vi "KE6517_Test.vi"(8 "error in (no error)":errorcluster, 11 "KE6517 in":refnum<class "KE6517.lvclass">) -> (0 "error out":errorcluster, 3 "KE6517 out":refnum<class "KE6517.lvclass">)   [LabVIEW 2013, in "KE6517.lvclass"]
uses:
  KE6517.lvclass
  <vilib>/Platform/TimedLoop/XDataNode/timing_clust.ctl
  <vilib>/Platform/TimedLoop/XDataNode/nitl_modes.ctl
  <vilib>/Platform/TimedLoop/XDataNode/wakeup.ctl
  InstrumentSetup.vi
  <vilib>/platform/TimedLoop/XDataNode/XDataNode.xnode
  <vilib>/Platform/TimedLoop/XDataNode/XDNodeRunTimeDep.lvlib
  InstrControl.lvclass
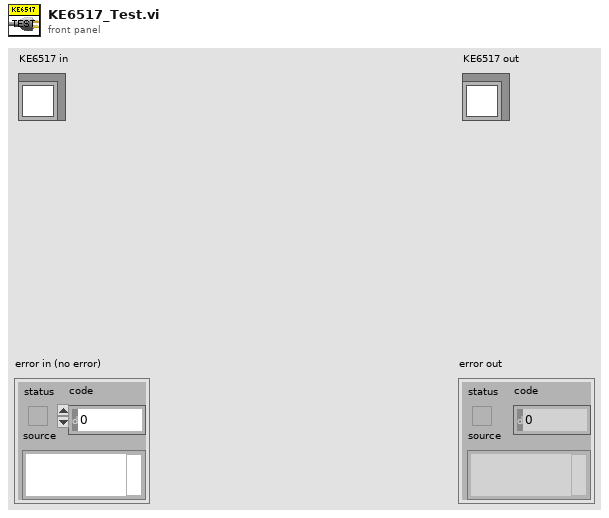
[diagram p1: front panel]
types:
  T1 = cluster{"KE 2410":cluster{"Instrument name":string, "address":refnum<visa-resource-name>, "Instrument type":u16}, "KE 6517":cluster{"Instrument name":string, "address":refnum<visa-resource-name>, "Instrument type":u16}, "KE 487":cluster{"Instrument name":string, "address":refnum<visa-resource-name>, "Instrument type":u16}, "KE 236":cluster{"Instrument name":string, "address":refnum<visa-resource-name>, "Instrument type":u16}, "WK 6440B":cluster{"Instrument name":string, "address":refnum<visa-resource-name>, "Instrument type":u16}, "WK 6425":cluster{"Instrument name":string, "address":refnum<visa-resource-name>, "Instrument type":u16}, "Pickering Matrix":cluster{"Instrument name":string, "address":refnum<visa-resource-name>, "Instrument type":u16}, "KE 2000":cluster{"Instrument name":string, "address":refnum<visa-resource-name>, "Instrument type":u16}, "KE3706A Switching":cluster{"Instrument name":string, "address":refnum<visa-resource-name>, "Instrument type":u16}}
  T2 = cluster{"Current Limit":u16, "KE6517":refnum<class "KE6517.lvclass">}
  T3 = typedef "XDNodeRunTimeDep.lvlib/timing_clust.ctl" = cluster{"Expected End [f-1]":u64, "Actual End [f-1]":u64, "Finished Late? [f-1]":bool, "Expected End [i-1]":u64, "Actual End [i-1]":u64, "Finished Late? [i-1]":bool, "Expected Start [i]":u64, "Actual Start [i]":u64, "Expected Start [f]":u64, "Actual Start [f]":u64, "Source Name":string, "Structure Name":string, "Period":i64, "Deadline":i64, "Offset":i64, "Start":i64, "Priority":i32, "Timeout":i32, "Mode":T4, "Wakeup Reason":T5, "Error":errorcluster, "Source Type":string, "Secondary Source Type":string, "Global End Time":u64, "Global Start Time":u64, "Frame Duration":u64, "Iteration Duration":u64, "Assigned CPU":i32, "I/O Scan Engine Mode":u32}
  T4 = typedef "XDNodeRunTimeDep.lvlib/nitl_modes.ctl" = enum32{"No Change", "Process missed periods, maintain original phase", "Discard missed periods, maintain original phase", "Process missed periods, ignore original phase", "Discard missed periods, ignore original phase"}
  T5 = typedef "XDNodeRunTimeDep.lvlib/wakeup.ctl" = enum32{"Normal", "Aborted", "Asynchronous wakeup", "Timing source error", "Timed loop error", "Timeout"}
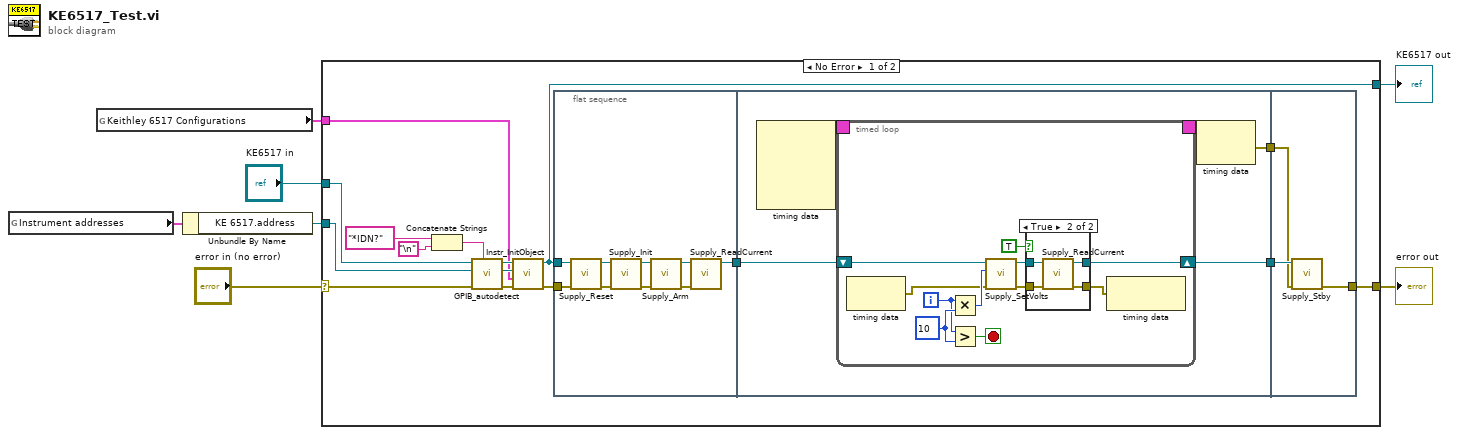
[diagram p0: block diagram]
diagram:
  n1 = global read "InstrumentSetup.vi" "Instrument addresses"() -> (w3:T1)
  n2 = global read "InstrumentSetup.vi" "Keithley 6517 Configurations"() -> (w1:T2)
  n3 = Unbundle By Name(w3) -> ("KE 6517.address"=w2:refnum<visa-resource-name>)
  n4 = case shown="No Error" "error in (no error)" {
    selector: "error in (no error)" -> [w18 w67]
    tunnel: [w20 w67] -> w6
    tunnel: [w16 w66] -> w4
    tunnel: "KE6517 in" -> [w14 w66]
    tunnel: w2 -> [w12 _]
    tunnel: w1 -> [w11 _]
    frame No Error {
      n5 = Concatenate Strings("*IDN?" ("regular expression"), "\n") -> (w9:string)
      n6 = call-dynamic "GPIB_autodetect.vi"("ID command"=w9, "error in (no error)"=w18, "Instrument address in"=w12, "InstrControl in"=w14) -> ("error out"=w19:errorcluster, "Instrument address out"=w13:refnum<visa-resource-name>, "InstrControl out"=w17:refnum<class "KE6517.lvclass">)  [unwired: 5 in]
      n7 = call-dynamic "Instr_InitObject.vi"("error in (no error)"=w19, "Instrument Configuration"=w11, "Instrument address"=w13, "KE6517 in"=w17) -> ("error out"=w15:errorcluster, "KE6517 out"=w16:refnum<class "KE6517.lvclass">)  [unwired: 6 in]
      n8 = flat-sequence {
        tunnel: w15 -> [w27]
        tunnel: w16 -> [w26]
        tunnel: [w24] -> w23
        tunnel: w23 -> [w37]
        tunnel: [w36] -> w22
        tunnel: [w33] -> w21
        tunnel: [w63] -> w20
        tunnel: w22 -> [w64]
        tunnel: w21 -> [w65]
        frame #0 {
          n9 = call-dynamic "Supply_Reset.vi"("error in (no error)"=w27, "SupplyControl in"=w26) -> ("error out"=w31:errorcluster, "SupplyControl out"=w25:refnum<class "KE6517.lvclass">)  [unwired: 8 in]
          n10 = call-dynamic "Supply_Init.vi"("error in (no error)"=w31, "SupplyControl in"=w25) -> ("error out"=w30:errorcluster, "SupplyControl out"=w32:refnum<class "KE6517.lvclass">)  [unwired: 8 in]
          n11 = call-dynamic "Supply_Arm.vi"("error in (no error)"=w30, "SupplyControl in"=w32) -> ("error out"=w28:errorcluster, "SupplyControl out"=w29:refnum<class "KE6517.lvclass">)  [unwired: 8 in]
          n12 = call-dynamic "Supply_ReadCurrent.vi"("error in (no error)"=w28, "SupplyControl in"=w29) -> ("SupplyControl out"=w24:refnum<class "KE6517.lvclass">)  [unwired: 7 in, 2 out]
        }
        frame #1 {
          n13 = node-c288() -> (w35:T3)  [unwired: 4 in]
          n14 = timed-loop {
            timing: w35 -> [_]
            timing-out: [_] -> w34
            shift-right: [w45] -> w33
            shift-left: w37 -> [w42]
            i -> [w47]
            stop <- w46 stop-if-true
            w48 = 10
            n15 = node-c288() -> (w40:errorcluster)  [unwired: 1 in]
            n16 = Multiply(x=w47, y=w48) -> (x*y=w41:i32)
            n17 = Greater?(x=w47, y=w48) -> (0:w46:bool)
            n18 = call-dynamic "Supply_SetVolts.vi"("error in (no error)"=w40, "Volts IN [V]"=w41, "KE6517 in"=w42) -> ("error out"=w38:errorcluster, "KE6517 out"=w39:refnum<class "KE6517.lvclass">)  [unwired: 6 in, 1 out]
            n19 = case shown="True" TRUE {
              tunnel: w38 -> [w50 w54]
              tunnel: w39 -> [w49 w53]
              tunnel: [w49 w52] -> w45
              tunnel: [w50 w51] -> w44
              frame False {
              }
              frame True {
                n20 = call-dynamic "Supply_ReadCurrent.vi"("error in (no error)"=w54, "SupplyControl in"=w53) -> ("error out"=w51:errorcluster, "SupplyControl out"=w52:refnum<class "KE6517.lvclass">)  [unwired: 7 in, 1 out]
              }
            }
            n21 = node-c288(w44) -> ()  [unwired: 1 out]
          }
          n22 = node-c288(w34) -> (w36:errorcluster)
        }
        frame #2 {
          n23 = call-dynamic "Supply_Stby.vi"("error in (no error)"=w64, "SupplyControl in"=w65) -> ("error out"=w63:errorcluster)  [unwired: 8 in, 1 out]
        }
      }
    }
    frame Error {
    }
  }
  "error out" <- w6
  "KE6517 out" <- w4
